vi "Get JSON.vi"(8 "error in (no error)":errorcluster, 11 "SLSC Session In":refnum<class "SLSC Interface.lvclass">) -> (0 "error out":errorcluster, 2 "capabilities":string, 3 "SLSC Session Out":refnum<class "SLSC Interface.lvclass">)   [LabVIEW 2016, in "SLSC Switch.lvlib" / "SLSC Switch.lvclass"]
uses:
  SLSC Switch.lvclass
  <vilib>/National Instruments/SLSC Local or Remote Interface/SLSC Interface Class/SLSC Interface.lvclass
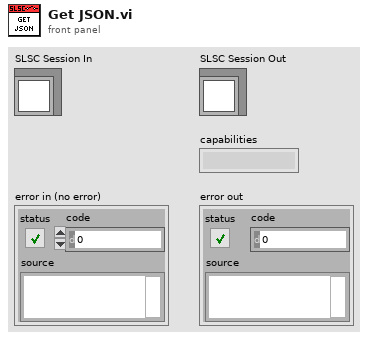
[diagram p1: front panel]
types:
  T1 = enum16{"open", "replace", "create", "open or create", "replace or create", "replace or create with confirmation"}
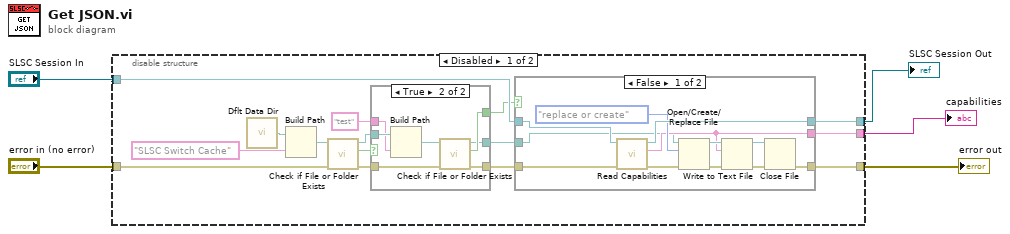
[diagram p0: block diagram]
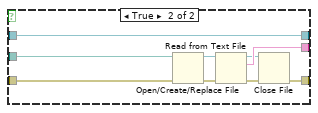
[diagram p2: hidden frame]
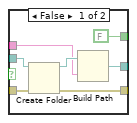
[diagram p3: hidden frame]
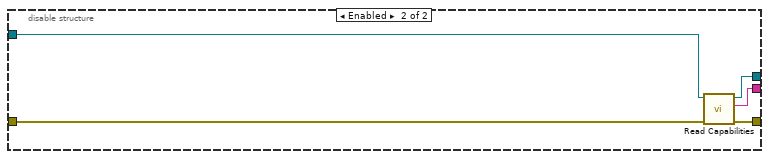
[diagram p4: hidden frame]
diagram:
  n1 = disable-structure shown="Disabled" {
    disable-tunnel: [w20 w57] -> w5
    disable-tunnel: [w17 w58] -> w4
    disable-tunnel: [w16 w59] -> w3
    disable-tunnel: "SLSC Session In" -> [w15 w60]
    disable-tunnel: "error in (no error)" -> [w7 w56]
    frame Disabled {
      n2 = call <vilib>:"Dflt Data Dir.vi"() -> ("App:Default Data Directory"=w9:path)
      n3 = Build Path(base path=w9, name or relative path="SLSC Switch Cache") -> (appended path=w11:path)
      n4 = call <vilib>:"Check if File or Folder Exists.vi"("error in (no error)"=w7, "path"=w11) -> ("error out"=w8:errorcluster, "file or folder exists?"=w6:bool, "dup path"=w12:path)  [unwired: 7 in]
      n5 = case shown="True" w6 {
        tunnel: w8 -> [w47 w53]
        tunnel: w12 -> [w48 w54]
        tunnel: [FALSE ("file or folder exists?") w52] -> w13
        tunnel: [w44 w51] -> w19
        tunnel: "test" ("name or relative path") -> [w45 w50]
        tunnel: [w42 w49] -> w18
        frame False {
          n6 = Create Folder(path (use dialog)=w48, error in=w47) -> (created path=w46:path, error out=w42:errorcluster)  [unwired: 1 in, 1 out]
          n7 = Build Path(base path=w46, name or relative path=w45) -> (appended path=w44:path)
        }
        frame True {
          n8 = Build Path(base path=w54, name or relative path=w50) -> (appended path=w55:path)
          n9 = call <vilib>:"Check if File or Folder Exists.vi"("error in (no error)"=w53, "path"=w55) -> ("error out"=w49:errorcluster, "file or folder exists?"=w52:bool, "dup path"=w51:path)  [unwired: 7 in]
        }
      }
      n10 = case shown="False" w13 {
        tunnel: w18 -> [w32 w37]
        tunnel: [w21 w35] -> w20
        tunnel: w15 -> [w31 w40]
        tunnel: [w30 w40] -> w16
        tunnel: [w26 w41] -> w17
        tunnel: w19 -> [w25 w33]
        frame False {
          n11 = call "Read Capabilities.vi"("error in (no error)"=w32, "SLSC NVMEM Session In"=w31) -> ("error out"=w22:errorcluster, "capabilities"=w26:string, "SLSC NVMEM Session Out"=w30:refnum<class "SLSC Interface.lvclass">)  [unwired: 7 in]
          n12 = Open/Create/Replace File(file path (use dialog)=w25, error in=w22, operation (0:open)=T1."replace or create") -> (refnum out=w27:refnum<file>, error out=w28:errorcluster)  [unwired: 3 in, 1 out]
          n13 = Write to Text File(file (use dialog)=w27, text=w26, error in=w28) -> (refnum out=w23:refnum<file>, error out=w24:errorcluster)  [unwired: 1 in, 1 out]
          n14 = Close File(refnum=w23, error in=w24) -> (error out=w21:errorcluster)  [unwired: 1 out]
        }
        frame True {
          n15 = Open/Create/Replace File(file path (use dialog)=w33, error in=w37) -> (refnum out=w38:refnum<file>, error out=w39:errorcluster)  [unwired: 4 in, 1 out]
          n16 = Read from Text File(file (use dialog)=w38, error in=w39) -> (refnum out=w34:refnum<file>, text=w41:string, error out=w36:errorcluster)  [unwired: 2 in, 1 out]
          n17 = Close File(refnum=w34, error in=w36) -> (error out=w35:errorcluster)  [unwired: 1 out]
        }
      }
    }
    frame Enabled {
      n18 = call "Read Capabilities.vi"("error in (no error)"=w56, "SLSC NVMEM Session In"=w60) -> ("error out"=w57:errorcluster, "capabilities"=w58:string, "SLSC NVMEM Session Out"=w59:refnum<class "SLSC Interface.lvclass">)  [unwired: 7 in]
    }
  }
  "error out" <- w5
  "capabilities" <- w4
  "SLSC Session Out" <- w3
